vi "SubVI_Downsample_EEG_rev2.vi"(8 "error in (no error)":errorcluster, 9 "Downsampling Rate":dbl, 10 "EEG Desired Frequency":dbl, 11 "Channel in":T2) -> (0 "error out":errorcluster, 3 "Channel out":T1)   [LabVIEW 2020]
uses:
  <extravilib>/ChannelInstances/Stream-a[.,.](dbl)/)Channel.ctl
  <extravilib>/ChannelInstances/Stream-a[.](dbl)/)Channel.ctl
  <extravilib>/ChannelInstances/Stream-a[.,.](dbl)/EndpointRead.vi
  <extravilib>/ChannelInstances/Stream-a[.](dbl)/Endpoint.vi
  Global 1.vi
  <extravilib>/ChannelInstances/Stream-a[.,.](dbl)/)Channel.vi
  <resource>/ChannelSupport/_ChannelSupport/WaitIfNeeded.vi
  <extravilib>/ChannelInstances/Stream-a[.](dbl)/)Channel.vi
  <extravilib>/ChannelInstances/Stream-a[.](dbl).lvlib
  <extravilib>/ChannelInstances/Stream-a[.,.](dbl).lvlib
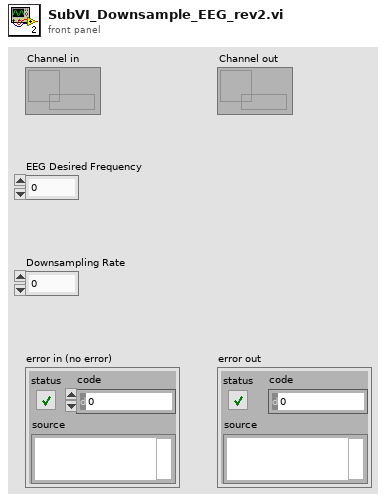
[diagram p1: front panel]
types:
  T1 = typedef "Stream-a[.](dbl).lvlib/)Channel.ctl" = refnum<queue>
  T2 = typedef "Stream-a[.,.](dbl).lvlib/)Channel.ctl" = refnum<queue>
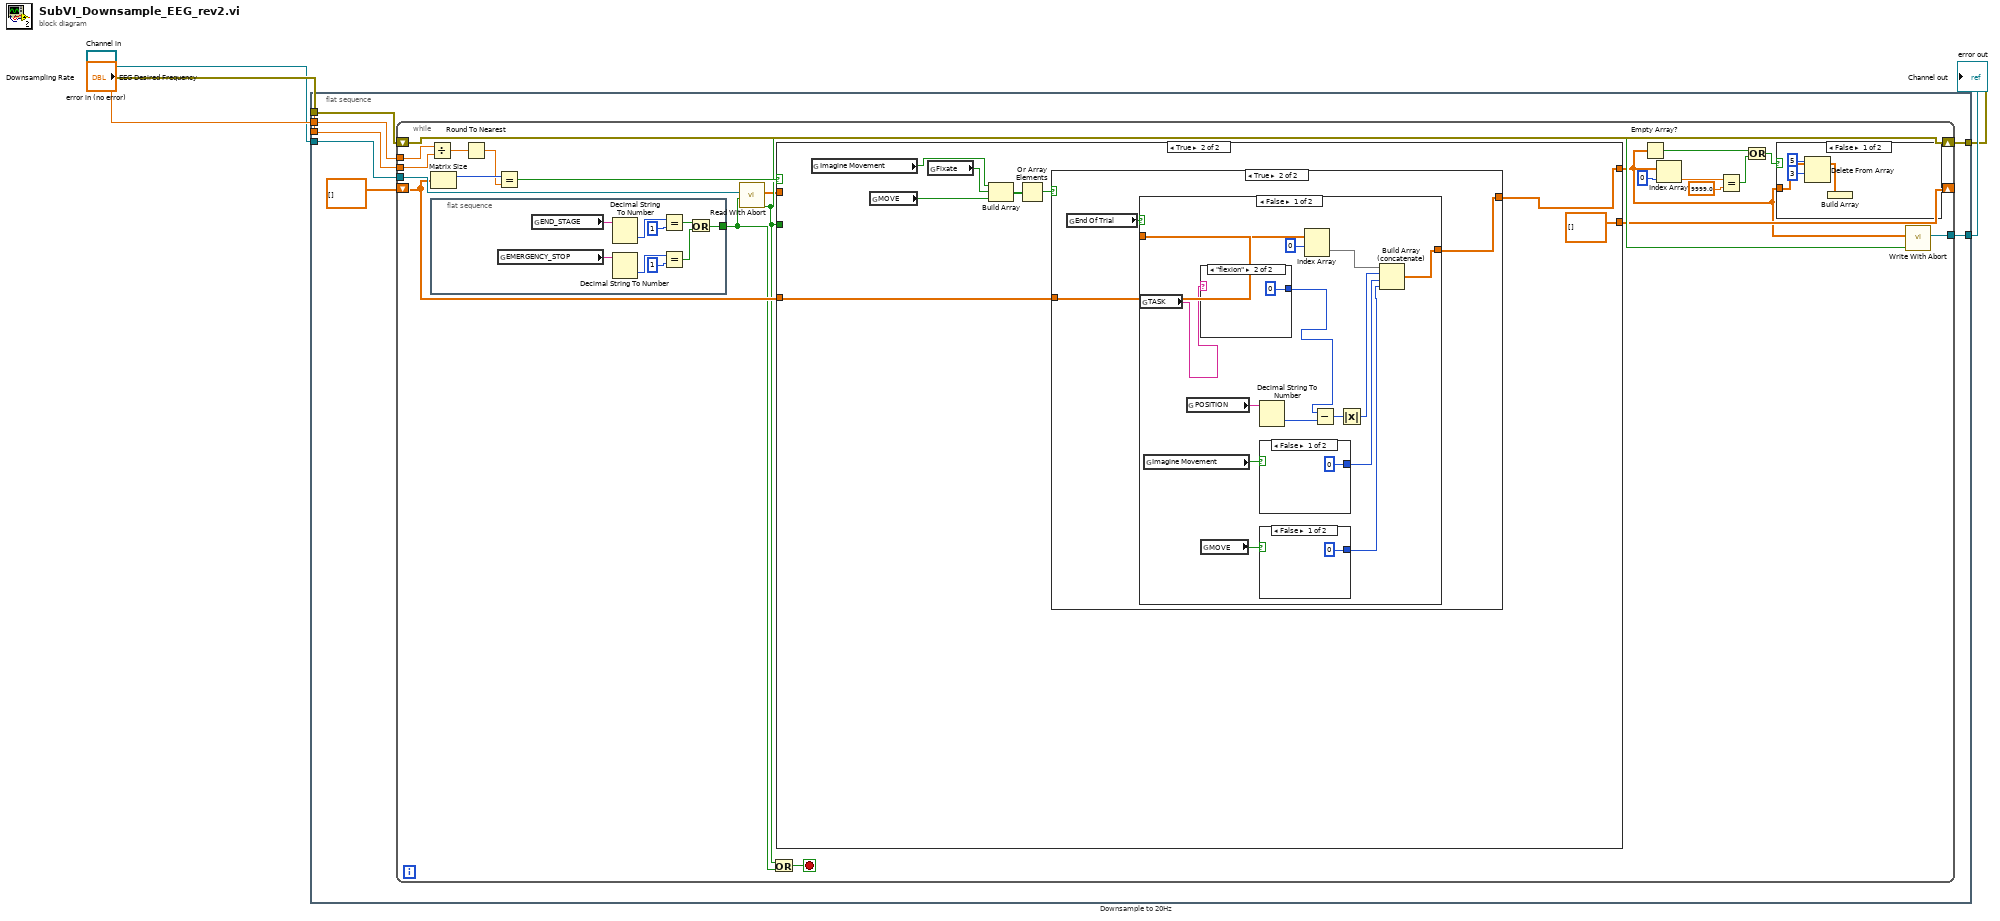
[diagram p0: block diagram]
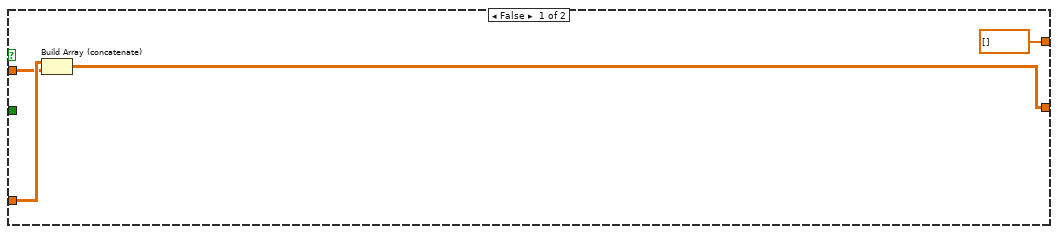
[diagram p3: hidden frame]
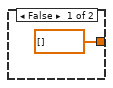
[diagram p4: hidden frame]
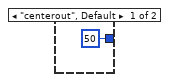
[diagram p5: hidden frame]
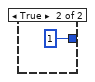
[diagram p6: hidden frame]
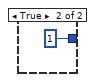
[diagram p7: hidden frame]
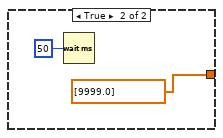
[diagram p8: hidden frame]
diagram:
  n1 = flat-sequence "Downsample to 20Hz" {
    tunnel: [w12] -> w2
    tunnel: [w11] -> w3
    tunnel: "error in (no error)" -> [w10]
    tunnel: "Channel in" -> [w9]
    tunnel: "EEG Desired Frequency" -> [w8]
    tunnel: "Downsampling Rate" -> [w7]
    frame #0 {
      n2 = while {
        tunnel: w9 -> [w35]
        shift-right: [w22] -> _
        shift-left: dbl[][] [] -> [w34]
        tunnel: w8 -> [w32]
        shift-right: [w27] -> w12
        shift-left: w10 -> [w27]
        tunnel: [w25] -> w11
        tunnel: w7 -> [w21]
        stop <- w28 stop-if-true
        n3 = Divide(x=w32, y=w21) -> (x/y=w31:dbl)
        n4 = Matrix Size(0:w34) -> (1:w33:i32)  [unwired: 1 out]
        n5 = flat-sequence {
          tunnel: [w40] -> w23
          frame #0 {
            n6 = global read "Global 1.vi" "EMERGENCY_STOP"() -> (w43:string)
            n7 = global read "Global 1.vi" "END_STAGE"() -> (w48:string)
            n8 = Decimal String To Number(string=w48) -> (number=w47:i32)  [unwired: 2 in, 1 out]
            n9 = Decimal String To Number(string=w43) -> (number=w45:i32)  [unwired: 2 in, 1 out]
            n10 = Equal?(x=w47, y=1) -> (x = y?=w41:bool)
            n11 = Equal?(x=w45, y=1) -> (x = y?=w42:bool)
            n12 = Or(x=w41, y=w42) -> (x .or. y?=w40:bool)
          }
        }
        n13 = Round To Nearest(number=w31) -> (nearest integer value=w30:dbl)
        n14 = Equal?(x=w33, y=w30) -> (x = y?=w29:bool)
        n15 = call <extravilib>:"Read With Abort.vi"("abort"=w23, "channel"=w35) -> ("element"=w24:dbl[][], "aborted?"=w26:bool)  [unwired: 4 in, 4 out]
        n16 = Or(x=w26, y=w23) -> (x .or. y?=w28:bool)
        n17 = case shown="True" w29 {
          tunnel: w34 -> [w52 w60]
          tunnel: w24 -> [w51 _]
          tunnel: [w50 dbl[][] []] -> w22
          tunnel: w26 -> [_ _]
          tunnel: [dbl[] [] w53] -> w14
          frame False {
            n18 = Build Array (concatenate)(w52, w51) -> (w50:dbl[][])
          }
          frame True {
            n19 = global read "Global 1.vi" "Imagine Movement"() -> (w57:bool)
            n20 = global read "Global 1.vi" "MOVE"() -> (w54:bool)
            n21 = global read "Global 1.vi" "Fixate"() -> (w56:bool)
            n22 = Build Array(w57, w56, w54) -> (w58:bool[])
            n23 = Or Array Elements(Boolean array=w58) -> (logical OR=w55:bool)
            n24 = case shown="True" w55 {
              tunnel: w60 -> [_ w64]
              tunnel: [dbl[] [] w63] -> w53
              frame False {
              }
              frame True {
                n25 = global read "Global 1.vi" "End Of Trial"() -> (w62:bool)
                n26 = case shown="False" w62 {
                  tunnel: w64 -> [w77 _]
                  tunnel: [w69 dbl[] [9999.0]] -> w63
                  frame False {
                    n27 = global read "Global 1.vi" "TASK"() -> (w65:string)
                    n28 = global read "Global 1.vi" "Imagine Movement"() -> (w74:bool)
                    n29 = global read "Global 1.vi" "POSITION"() -> (w75:string)
                    n30 = case shown="\"flexion\"" w65 {
                      tunnel: [50 0] -> w66
                      frame "centerout", Default {
                      }
                      frame "flexion" {
                      }
                    }
                    n31 = global read "Global 1.vi" "MOVE"() -> (w76:bool)
                    n32 = Decimal String To Number(string=w75) -> (number=w73:i32)  [unwired: 2 in, 1 out]
                    n33 = case shown="False" w74 {
                      tunnel: [0 1] -> w70
                      frame False {
                      }
                      frame True {
                      }
                    }
                    n34 = case shown="False" w76 {
                      tunnel: [0 1] -> w68
                      frame False {
                      }
                      frame True {
                      }
                    }
                    n35 = Index Array(array=w77, index (row)=0) -> (element=w67:dbl[])  [unwired: 1 in]
                    n36 = Subtract(x=w66, y=w73) -> (x-y=w72:i32)
                    n37 = Absolute Value(x=w72) -> (abs(x)=w71:i32)
                    n38 = Build Array (concatenate)(w67, w71, w70, w68) -> (w69:dbl[])
                  }
                  frame True {
                    n39 = Wait (ms)(milliseconds to wait=u32 50) -> ()  [unwired: 1 out]
                  }
                }
              }
            }
          }
        }
        n40 = Empty Array?(array=w14) -> (empty?=w16:bool)
        n41 = Index Array(array=w14, index=0) -> (element=w19:dbl)
        n42 = Equal?(x=w19, y=9999.0) -> (x = y?=w17:bool)
        n43 = Or(x=w16, y=w17) -> (x .or. y?=w15:bool)
        n44 = case shown="False" w15 {
          tunnel: w14 -> [w39 _]
          frame False {
            n45 = Delete From Array(array=w39, length=3, index=5) -> (array with subset deleted=w36:dbl[])  [unwired: 1 out]
            n46 = Build Array(w36) -> ()  [unwired: 1 out]
          }
          frame True {
          }
        }
        n47 = call <extravilib>:"Write With Abort.vi"("abort"=w26, "element"=w14) -> ("channel"=w25:T1)  [unwired: 6 in, 3 out]
      }
    }
  }
  "Channel out" <- w3
  "error out" <- w2
